vi "TDMS Copy Group.vi"(7 "group name":string, 8 "error in":errorcluster, 10 "tdms dest in":refnum<k34>, 11 "tdms source in":refnum<k34>) -> (0 "error out":errorcluster, 2 "tdms dest out":refnum<k34>, 3 "tdms source out":refnum<k34>)   [LabVIEW 2011]
doc: "Copies the properties and the channels of the group from the source file to the destination file. Existing properties become overwritten. New channel data is appended to the old one if present."
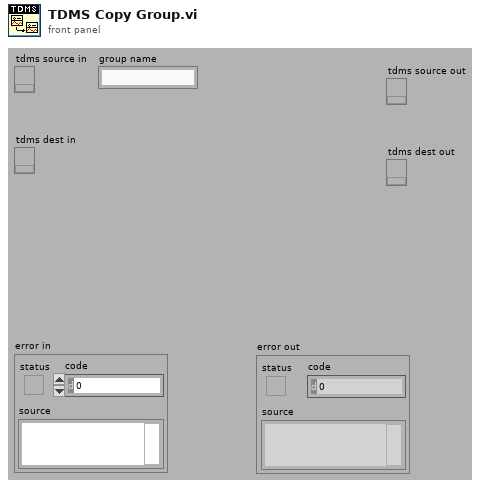
[diagram p1: front panel]
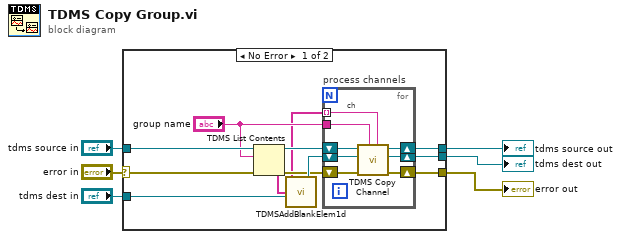
[diagram p0: block diagram]
diagram:
  n1 = case shown="No Error" "error in" {
    selector: "error in" -> [w8 w26]
    tunnel: "tdms dest in" -> [w17 w27]
    tunnel: "tdms source in" -> [w16 w28]
    tunnel: [w11 w28] -> w4
    tunnel: [w10 w27] -> w3
    tunnel: [w9 w26] -> w2
    frame No Error {
      n2 = TDMS List Contents(4:w8, 6:"group name", 7:w16) -> (0:w15:errorcluster, 1:w7:string[], 3:w14:refnum<k34>)  [unwired: 1 out]
      n3 = call <vilib>:"TDMSAddBlankElem1d.vi"("input string array"=w7) -> ("output string array with blank element at the beginning"=w12:string[])
      n4 = for "process channels" {
        tunnel: "group name" -> [w19]
        tunnel: w12 -> [w18] mode=indexing
        shift-right: [w24] -> w9
        shift-left: w15 -> [w21]
        shift-right: [w23] -> w10
        shift-left: w17 -> [w25]
        shift-right: [w22] -> w11
        shift-left: w14 -> [w20]
        # "ch"
        n5 = call "TDMS Copy Channel.vi"("channel name"=w18, "group name"=w19, "error in"=w21, "tdms dest in"=w25, "tdms source in"=w20) -> ("error out"=w24:errorcluster, "tdms dest out"=w23:refnum<k34>, "tdms source out"=w22:refnum<k34>)  [unwired: 4 out]
      }
    }
    frame Error {
    }
  }
  "error out" <- w2
  "tdms source out" <- w4
  "tdms dest out" <- w3
